vi "DRWM_SSF.vi"(0 "反应性in":dbl[](array[numeric]), 5 "SSF因子":cluster{"x":dbl, "y":dbl}[][](array[cluster]), 7 "P2信号":dbl[](array[numeric]), 9 "时间步长":sgl, 11 "通量in":dbl[](array[numeric]), 12 "首次调用？":bool) -> (4 "上下段通量索引":u16[](array[numeric]), 6 "DRWM开":bool, 8 "P2信号out":dbl[](array[numeric]), 10 "通量out":dbl[](array[numeric]), 14 "棒限":dbl[](array[numeric]), 15 "刻棒棒位":dbl)   [LabVIEW 2020]
uses:
  <vilib>/Analysis/baseanly.llb/Mean (DBL).vi
  <vilib>/Analysis/NI_AALBase.lvlib
panel:
  in  "DSF2合1":bool
  in  "上下段比值":dbl=0.0001 min=0.0001 max=100.0 step=0.0001 format="%0.2f"
  in  "修正因子选择":u16(ring) items=["C1", "C2", "C3", "C4", "C5", "C6", "C7", "C8", "C9", "10"]
  out "因子说明":string caption="修正因子文件说明："
  in  "因子棒名":string[](array[string])
  in  "底部棒位 (步)":dbl=5.0
  in  "触发准备":bool
  out "触发量稳定值":dbl
  in  "反应性触发选择":u16(ring) items=["电流1", "电流2"]
  out "触发量散度 (%)":dbl
  in  "触发量容限 (%)":dbl=10.0
  in  "反应性暂存":dbl[](array[numeric])
  in  "棒位暂存":dbl[](array[numeric])
  in  "触发方式":u16(ring)=3 items=["手动触发启动", "反应性触发启动", "棒位触发启动", "实时棒位无需触发"]
  in  "顶部棒位 (步)":dbl=225.0
  in  "棒速 (步/分钟)":dbl=72.0
  out "DRWM控制棒":dbl(slide) min=0.0 max=225.0 scale=0.0..225.0
  in  "开关":bool
  in  "上部探测器选择":u16(ring) items=["电流1", "电流2"]
  in  "下部探测器选择":u16(ring)=1 items=["电流1", "电流2"]
  in  "通量名称":string[](array[string])
  in  "P2名称":string[](array[string])
  in  "控制棒选择":i32(ring) items=["棒位D", "棒位C", "电压6"]
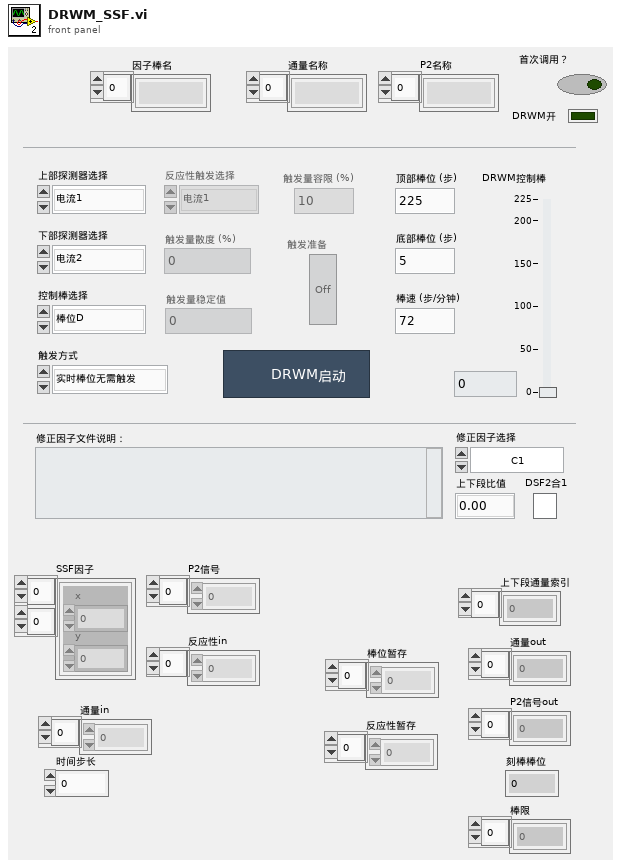
[diagram p1: front panel]
types:
  T1 = enum8{"Enabled", "Disabled", "Disabled and Grayed Out"}
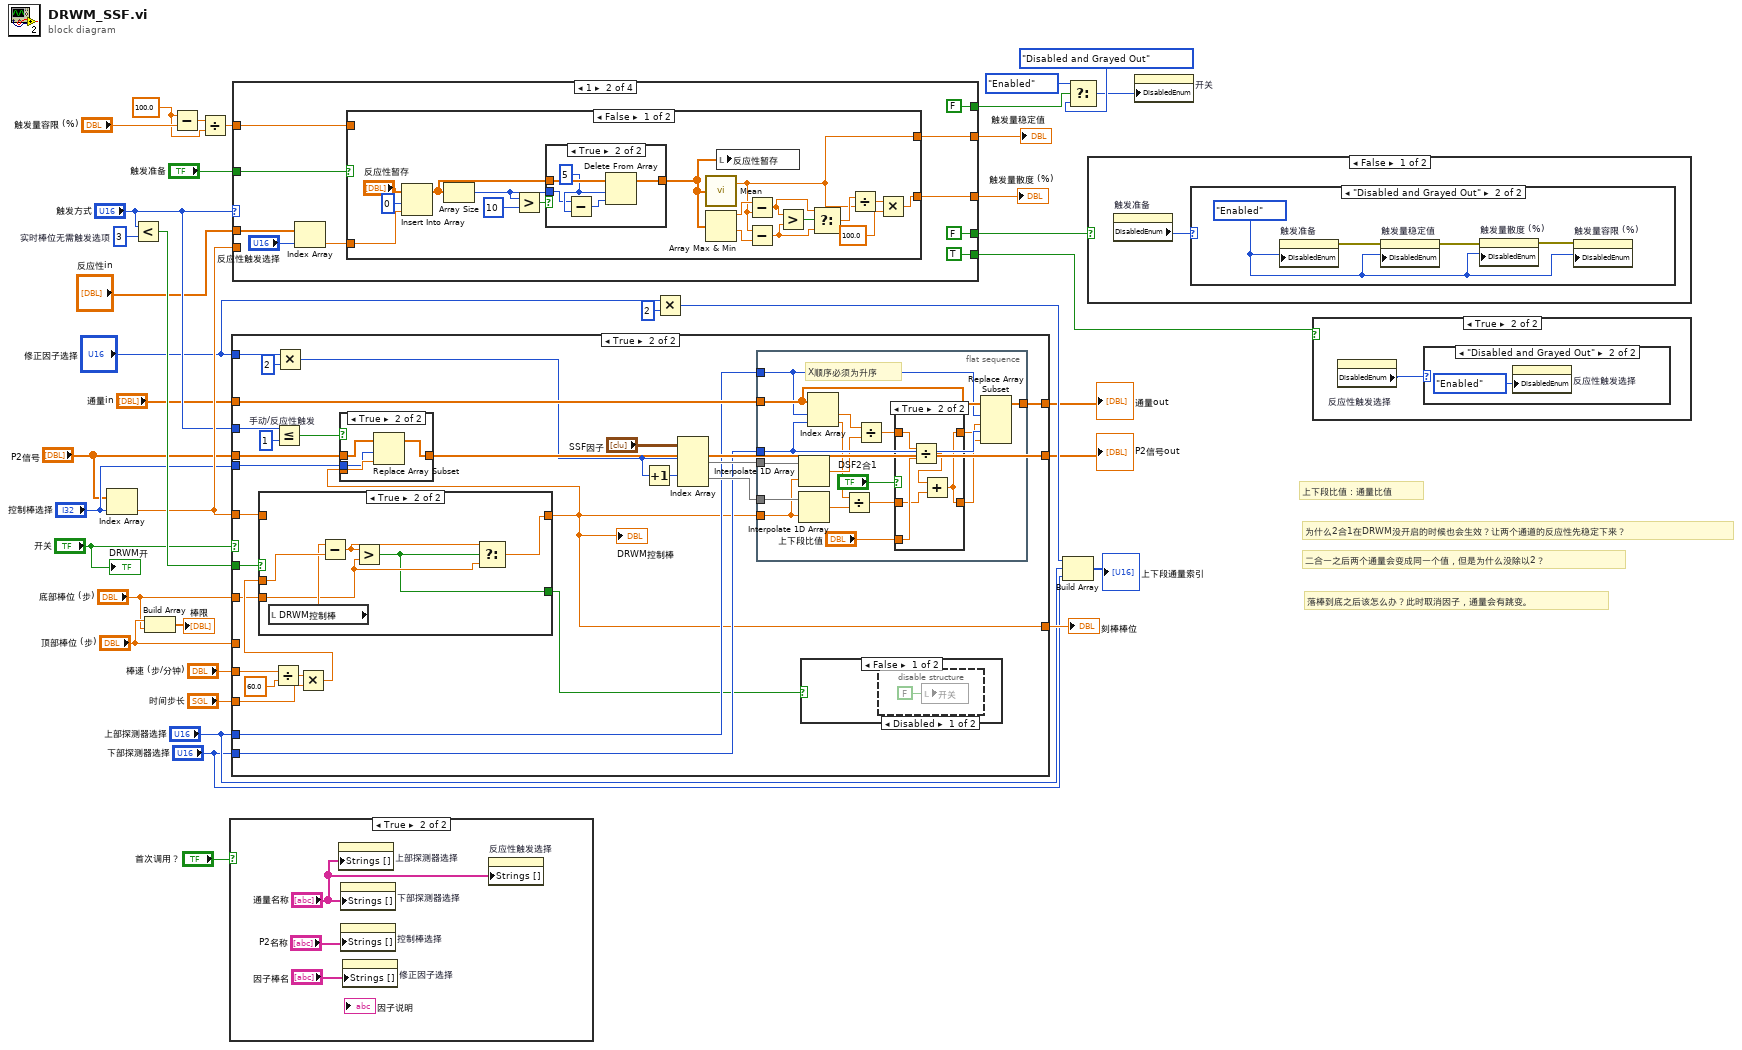
[diagram p0: block diagram]
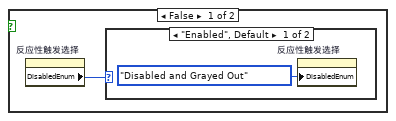
[diagram p2: hidden frame]
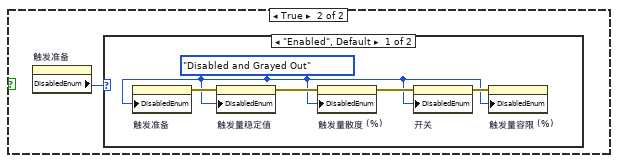
[diagram p6: hidden frame]
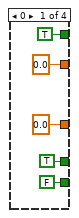
[diagram p8: hidden frame]
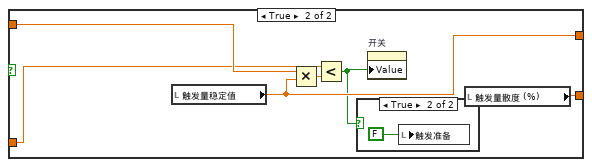
[diagram p10: hidden frame]
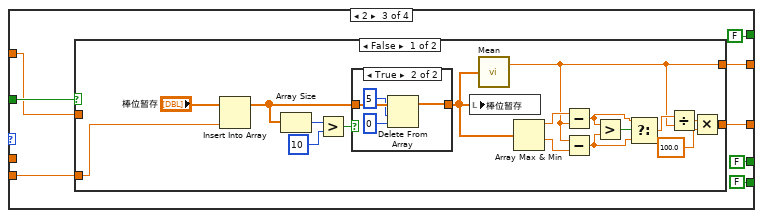
[diagram p12: hidden frame]
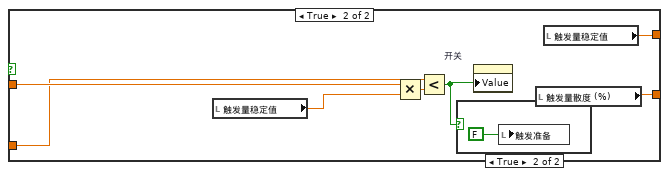
[diagram p14: hidden frame]
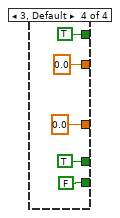
[diagram p16: hidden frame]
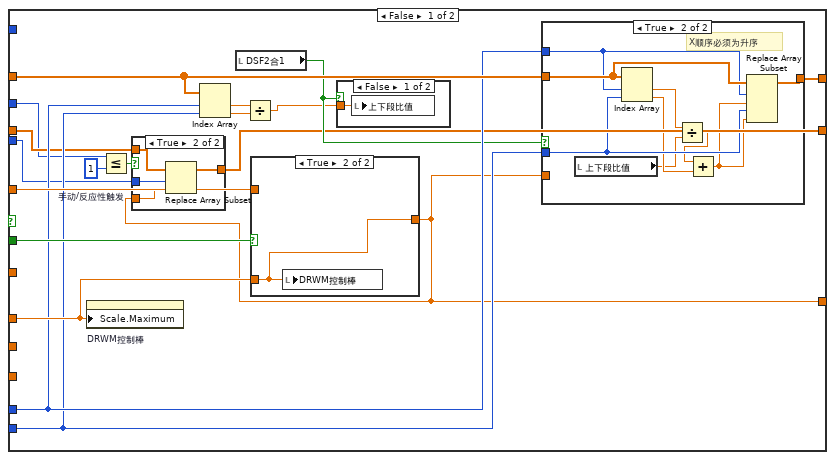
[diagram p17: hidden frame]
diagram:
  w31 = 100.0 ("x")
  w34 = u16 3  # 实时棒位无需触发选项
  # "落棒到底之后该怎么办？此时取消因子，通量会有跳变。"
  # "二合一之后两个通量会变成同一个值，但是为什么没除以2？"
  # "为什么2合1在DRWM没开启的时候也会生效？让两个通道的反应性先稳定下来？"
  # "上下段比值：通量比值"
  n1 = Index Array(array="P2信号", index="控制棒选择") -> (element=w30:dbl)
  n2 = Less?(x="触发方式", y=w34) -> (x < y?=w35:bool)
  n3 = Build Array("顶部棒位 (步)", "底部棒位 (步)") -> (→"棒限":dbl[])
  n4 = Subtract(x=w31, y="触发量容限 (%)") -> (x-y=w32:dbl)
  n5 = Divide(x=w32, y=w31) -> (x/y=w29:dbl)
  n6 = case shown="True" "首次调用？" {
    frame False {
    }
    frame True {
      n7 = property on="上部探测器选择" class="Ring (strict)"("Strings []"="通量名称") -> ()  [unwired: 2 in, 2 out]
      n8 = property on="下部探测器选择" class="Ring (strict)"("Strings []"="通量名称") -> ()  [unwired: 2 in, 2 out]
      n9 = property on="控制棒选择" class="Ring (strict)"("Strings []"="P2名称") -> ()  [unwired: 2 in, 2 out]
      n10 = property on="修正因子选择" class="Ring (strict)"("Strings []"="因子棒名") -> ()  [unwired: 2 in, 2 out]
      n11 = property on="反应性触发选择" class="Ring (strict)"("Strings []"="通量名称") -> ()  [unwired: 2 in, 2 out]
    }
  }
  n12 = case shown="True" "开关" {
    tunnel: "通量in" -> [w53 w103]
    tunnel: [w52 w102] -> w9
    tunnel: "棒速 (步/分钟)" -> [_ w98]
    tunnel: "时间步长" -> [_ w94]
    tunnel: "顶部棒位 (步)" -> [w56 _]
    tunnel: w35 -> [w57 w96]
    tunnel: w30 -> [w58 w95]
    tunnel: [w45 w78] -> w27
    tunnel: "P2信号" -> [w44 w88]
    tunnel: [w43 w87] -> w11
    tunnel: "触发方式" -> [w42 w91]
    tunnel: "控制棒选择" -> [w46 w86]
    tunnel: "底部棒位 (步)" -> [_ w85]
    tunnel: "修正因子选择" -> [_ w84]
    tunnel: "上部探测器选择" -> [w51 w80]
    tunnel: "下部探测器选择" -> [w50 w79]
    frame False {
      w48 = u16 1  # 手动/反应性触发
      n13 = property on="DRWM控制棒" class="Slide (strict)"("Scale.Maximum"=w56) -> ()  [unwired: 2 in, 2 out]
      n14 = Less Or Equal?(x=w42, y=w48) -> (x <= y?=w47:bool)
      n15 = Index Array(array=w53, index #1=w51, index #2=w50) -> (element #1=w55:dbl, element #2=w54:dbl)
      n16 = local read "DSF2合1"() -> (w49:bool)
      n17 = Divide(x=w55, y=w54) -> (x/y=w41:dbl)
      n18 = case shown="True" w57 {
        tunnel: [w75 w76] -> w45
        tunnel: w58 -> [w75 _]
        tunnel: w56 -> [_ w76]
        frame False {
          n19 = local write "DRWM控制棒"(w75) -> ()
        }
        frame True {
          n20 = local write "DRWM控制棒"(w76) -> ()
        }
      }
      n21 = case shown="True" w47 {
        tunnel: w44 -> [w59 w63]
        tunnel: [w59 w62] -> w43
        tunnel: w45 -> [_ w61]
        tunnel: w46 -> [_ w60]
        frame False {
        }
        frame True {
          n22 = Replace Array Subset(array=w63, new element=w61, index=w60) -> (w62:dbl[])
        }
      }
      n23 = case shown="False" w49 {
        tunnel: w41 -> [w74 _]
        frame False {
          n24 = local write "上下段比值"(w74) -> ()
        }
        frame True {
        }
      }
      n25 = case shown="True" w49 {
        tunnel: w53 -> [w64 w73]
        tunnel: [w64 w72] -> w52
        tunnel: w45 -> [_ _]
        tunnel: w51 -> [_ w71]
        tunnel: w50 -> [_ w70]
        frame False {
        }
        frame True {
          # "X顺序必须为升序"
          n26 = local read "上下段比值"() -> (w66:dbl)
          n27 = Index Array(array=w73, index #1=w71, index #2=w70) -> (element #1=w67:dbl, element #2=w68:dbl)
          n28 = Divide(x=w67, y=w66) -> (x/y=w65:dbl)
          n29 = Add(x=w65, y=w68) -> (x+y=w69:dbl)
          n30 = Replace Array Subset(array=w73, new element #1=w69, index #1=w71, new element #2=w69, index #2=w70) -> (w72:dbl[])
        }
      }
    }
    frame True {
      w90 = u16 1  # 手动/反应性触发
      n31 = Divide(x=w98, y=60.0) -> (x/y=w93:dbl)
      n32 = Less Or Equal?(x=w91, y=w90) -> (x <= y?=w89:bool)
      n33 = Multiply(x=w84, y=u16 2) -> (x*y=w81:u16)
      n34 = Multiply(x=w93, y=w94) -> (x*y=w92:dbl)
      n35 = case shown="True" w96 {
        tunnel: w95 -> [w134 _]
        tunnel: [w134 w137] -> w78
        tunnel: w92 -> [_ w142]
        tunnel: w85 -> [w136 w139]
        tunnel: [w135 w138] -> w77
        frame False {
          n36 = Greater?(x=w134, y=w136) -> (0:w135:bool)
        }
        frame True {
          n37 = local read "DRWM控制棒"() -> (w140:dbl)
          n38 = Subtract(x=w140, y=w142) -> (x-y=w141:dbl)
          n39 = Greater?(x=w141, y=w139) -> (0:w138:bool)
          n40 = Select(t=w141, s=w138, f=w139) -> (s? t:f=w137:dbl)
        }
      }
      "DRWM控制棒" <- w78
      n41 = case shown="True" w89 {
        tunnel: w88 -> [w129 w133]
        tunnel: [w129 w132] -> w87
        tunnel: w78 -> [_ w131]
        tunnel: w86 -> [_ w130]
        frame False {
        }
        frame True {
          n42 = Replace Array Subset(array=w133, new element=w131, index=w130) -> (w132:dbl[])
        }
      }
      n43 = Increment(x=w81) -> (x+1=w82:u16)
      n44 = Index Array(array="SSF因子", index (row) #1=w81, index (row) #2=w82) -> (element #1=w100:cluster{"x":dbl, "y":dbl}[], element #2=w99:cluster{"x":dbl, "y":dbl}[])  [unwired: 2 in]
      n45 = flat-sequence {
        tunnel: w103 -> [w121]
        tunnel: [w120] -> w102
        tunnel: w100 -> [w119]
        tunnel: w99 -> [w118]
        tunnel: w80 -> [w117]
        tunnel: w79 -> [w116]
        tunnel: w78 -> [w115]
        frame #0 {
          # "X顺序必须为升序"
          n46 = Interpolate 1D Array(1:w115, 2:w119) -> (0:w113:dbl)
          n47 = Interpolate 1D Array(1:w115, 2:w118) -> (0:w112:dbl)
          n48 = Index Array(array=w121, index #1=w117, index #2=w116) -> (element #1=w114:dbl, element #2=w111:dbl)
          n49 = Divide(x=w111, y=w112) -> (x/y=w109:dbl)
          n50 = Divide(x=w114, y=w113) -> (x/y=w110:dbl)
          n51 = case shown="True" "DSF2合1" {
            tunnel: w110 -> [w123 w128]
            tunnel: w109 -> [w122 w126]
            tunnel: [w122 w124] -> w108
            tunnel: [w123 w124] -> w107
            tunnel: "上下段比值" -> [_ w127]
            frame False {
            }
            frame True {
              n52 = Divide(x=w128, y=w127) -> (x/y=w125:dbl)
              n53 = Add(x=w125, y=w126) -> (x+y=w124:dbl)
            }
          }
          n54 = Replace Array Subset(array=w121, new element #1=w107, index #1=w117, new element #2=w108, index #2=w116) -> (w120:dbl[])
        }
      }
      n55 = case shown="False" w77 {
        frame False {
          n56 = disable-structure shown="Disabled" {
            frame Disabled {
              n57 = local write "开关"(FALSE ("开关")) -> ()
            }
            frame Enabled {
            }
          }
        }
        frame True {
        }
      }
    }
  }
  "通量out" <- w9
  "刻棒棒位" <- w27
  "P2信号out" <- w11
  n58 = case shown="1" "触发方式" {
    tunnel: w30 -> [_ _ w196 _]
    tunnel: w29 -> [_ w151 w193 _]
    tunnel: "反应性in" -> [_ w153 _ _]
    tunnel: [0.0 ("触发量散度%") w157 w195 0.0] -> w28
    tunnel: [0.0 ("mean") w156 w192 0.0 ("触发量稳定值")] -> w26
    tunnel: "触发准备" -> [_ w152 w194 _]
    tunnel: [TRUE FALSE FALSE TRUE] -> w24
    tunnel: [FALSE TRUE FALSE FALSE] -> w23
    tunnel: [TRUE FALSE FALSE TRUE] -> w4
    frame 0 {
    }
    frame 1 {
      n59 = Index Array(array=w153, index="反应性触发选择") -> (element=w154:dbl)
      n60 = case shown="False" w152 {
        tunnel: [w160 w187] -> w157
        tunnel: [w159 w185] -> w156
        tunnel: w154 -> [w158 w182]
        tunnel: w151 -> [_ w183]
        frame False {
          n61 = Insert Into Array(array="反应性暂存", index=0 ("索引"), new element=w158) -> (w172:dbl[])
          n62 = Array Size(array=w172) -> (size(s)=w170:i32)
          n63 = Greater?(x=w170, y=10) -> (0:w175:bool)
          n64 = case shown="True" w175 {
            tunnel: w172 -> [w176 w180]
            tunnel: [w176 w181] -> w171
            tunnel: w170 -> [_ w178]
            frame False {
            }
            frame True {
              w179 = 5 ("长度")
              n65 = Subtract(x=w178, y=w179) -> (x-y=w177:i32)
              n66 = Delete From Array(array=w180, length=w179, index=w177) -> (array with subset deleted=w181:dbl[])  [unwired: 1 out]
            }
          }
          n67 = call-poly <vilib>:"Mean.vi"("X"=w171) -> ("mean"=w159:dbl)  [unwired: 1 out]
          n68 = Array Max & Min(array=w171) -> (max value=w168:dbl, min value=w167:dbl)  [unwired: 2 out]
          n69 = local write "反应性暂存"(w171) -> ()
          n70 = Subtract(x=w168, y=w159) -> (x-y=w165:dbl)
          n71 = Subtract(x=w159, y=w167) -> (x-y=w164:dbl)
          n72 = Greater?(x=w165, y=w164) -> (0:w166:bool)
          n73 = Select(t=w165, s=w166, f=w164) -> (s? t:f=w163:dbl)
          n74 = Divide(x=w163, y=w159) -> (x/y=w162:dbl)
          n75 = Multiply(x=w162, y=100.0) -> (x*y=w160:dbl)
        }
        frame True {
          n76 = local read "触发量稳定值"() -> (w185:dbl)
          n77 = Multiply(x=w183, y=w185) -> (x*y=w186:dbl)
          n78 = Less?(x=w182, y=w186) -> (x < y?=w184:bool)
          n79 = case shown="True" w184 {
            frame False {
            }
            frame True {
              n80 = local write "触发准备"(FALSE ("触发准备")) -> ()
            }
          }
          n81 = property on="开关" class="Bool (strict)"("Value"=w184) -> ()  [unwired: 2 in, 2 out]
          n82 = local read "触发量散度 (%)"() -> (w187:dbl)
        }
      }
    }
    frame 2 {
      n83 = case shown="False" w194 {
        tunnel: w196 -> [w208 w219]
        tunnel: [w198 w224] -> w195
        tunnel: w193 -> [_ w222]
        tunnel: [w197 w220] -> w192
        frame False {
          n84 = Insert Into Array(array="棒位暂存", new element=w208) -> (w212:dbl[])  [unwired: 1 in]
          n85 = Array Size(array=w212) -> (size(s)=w210:i32)
          n86 = Greater?(x=w210, y=10) -> (0:w213:bool)
          n87 = case shown="True" w213 {
            tunnel: w212 -> [w214 w217]
            tunnel: [w214 w218] -> w204
            frame False {
            }
            frame True {
              n88 = Delete From Array(array=w217, length=5 ("长度"), index=0 ("索引")) -> (array with subset deleted=w218:dbl[])  [unwired: 1 out]
            }
          }
          n89 = local write "棒位暂存"(w204) -> ()
          n90 = call-poly <vilib>:"Mean.vi"("X"=w204) -> ("mean"=w197:dbl)  [unwired: 1 out]
          n91 = Array Max & Min(array=w204) -> (max value=w203:dbl, min value=w207:dbl)  [unwired: 2 out]
          n92 = Subtract(x=w203, y=w197) -> (x-y=w202:dbl)
          n93 = Subtract(x=w197, y=w207) -> (x-y=w205:dbl)
          n94 = Greater?(x=w202, y=w205) -> (0:w206:bool)
          n95 = Select(t=w202, s=w206, f=w205) -> (s? t:f=w199:dbl)
          n96 = Divide(x=w199, y=w197) -> (x/y=w201:dbl)
          n97 = Multiply(x=w201, y=100.0) -> (x*y=w198:dbl)
        }
        frame True {
          n98 = local read "触发量稳定值"() -> (w223:dbl)
          n99 = Multiply(x=w222, y=w223) -> (x*y=w225:dbl)
          n100 = Less?(x=w219, y=w225) -> (x < y?=w221:bool)
          n101 = case shown="True" w221 {
            frame False {
            }
            frame True {
              n102 = local write "触发准备"(FALSE ("触发准备")) -> ()
            }
          }
          n103 = property on="开关" class="Bool (strict)"("Value"=w221) -> ()  [unwired: 2 in, 2 out]
          n104 = local read "触发量散度 (%)"() -> (w224:dbl)
          n105 = local read "触发量稳定值"() -> (w220:dbl)
        }
      }
    }
    frame 3, Default {
    }
  }
  "触发量散度 (%)" <- w28
  "触发量稳定值" <- w26
  n106 = Multiply(x="修正因子选择", y=u16 2) -> (x*y=w13:u16)
  n107 = Build Array(w13, "上部探测器选择", "下部探测器选择") -> (→"上下段通量索引":u16[])
  n108 = Select(t=T1."Enabled" ("禁用"), s=w4, f=T1."Disabled and Grayed Out" ("禁用")) -> (s? t:f=w1:T1)
  n109 = case shown="False" w24 {
    frame False {
      n110 = property on="触发准备" class="Bool (strict)"() -> ("DisabledEnum"=w232:T1)  [unwired: 2 in, 2 out]
      n111 = case shown="\"Disabled and Grayed Out\"" w232 {
        frame "Enabled", Default {
        }
        frame "Disabled and Grayed Out" {
          w234 = T1."Enabled" ("禁用")
          n112 = property on="触发准备" class="Bool (strict)"("DisabledEnum"=w234) -> (error out=w236:errorcluster)  [unwired: 2 in, 1 out]
          n113 = property on="触发量稳定值" class="DigNum (strict)"(error in=w236, "DisabledEnum"=w234) -> (error out=w235:errorcluster)  [unwired: 1 in, 1 out]
          n114 = property on="触发量散度 (%)" class="DigNum (strict)"(error in=w235, "DisabledEnum"=w234) -> (error out=w233:errorcluster)  [unwired: 1 in, 1 out]
          n115 = property on="触发量容限 (%)" class="DigNum (strict)"(error in=w233, "DisabledEnum"=w234) -> ()  [unwired: 1 in, 2 out]
        }
      }
    }
    frame True {
      n116 = property on="触发准备" class="Bool (strict)"() -> ("DisabledEnum"=w237:T1)  [unwired: 2 in, 2 out]
      n117 = case shown="\"Enabled\", Default" w237 {
        frame "Enabled", Default {
          w238 = T1."Disabled and Grayed Out" ("禁用")
          n118 = property on="触发准备" class="Bool (strict)"("DisabledEnum"=w238) -> (error out=w241:errorcluster)  [unwired: 2 in, 1 out]
          n119 = property on="触发量稳定值" class="DigNum (strict)"(error in=w241, "DisabledEnum"=w238) -> (error out=w242:errorcluster)  [unwired: 1 in, 1 out]
          n120 = property on="触发量散度 (%)" class="DigNum (strict)"(error in=w242, "DisabledEnum"=w238) -> (error out=w240:errorcluster)  [unwired: 1 in, 1 out]
          n121 = property on="开关" class="Bool (strict)"(error in=w240, "DisabledEnum"=w238) -> (error out=w239:errorcluster)  [unwired: 1 in, 1 out]
          n122 = property on="触发量容限 (%)" class="DigNum (strict)"(error in=w239, "DisabledEnum"=w238) -> ()  [unwired: 1 in, 2 out]
        }
        frame "Disabled and Grayed Out" {
        }
      }
    }
  }
  n123 = property on="开关" class="Bool (strict)"("DisabledEnum"=w1) -> ()  [unwired: 2 in, 2 out]
  n124 = case shown="True" w23 {
    frame False {
      n125 = property on="反应性触发选择" class="Ring (strict)"() -> ("DisabledEnum"=w243:T1)  [unwired: 2 in, 2 out]
      n126 = case shown="\"Enabled\", Default" w243 {
        frame "Enabled", Default {
          n127 = property on="反应性触发选择" class="Ring (strict)"("DisabledEnum"=T1."Disabled and Grayed Out" ("禁用")) -> ()  [unwired: 2 in, 2 out]
        }
        frame "Disabled and Grayed Out" {
        }
      }
    }
    frame True {
      n128 = property on="反应性触发选择" class="Ring (strict)"() -> ("DisabledEnum"=w245:T1)  [unwired: 2 in, 2 out]
      n129 = case shown="\"Disabled and Grayed Out\"" w245 {
        frame "Enabled", Default {
        }
        frame "Disabled and Grayed Out" {
          n130 = property on="反应性触发选择" class="Ring (strict)"("DisabledEnum"=T1."Enabled" ("禁用")) -> ()  [unwired: 2 in, 2 out]
        }
      }
    }
  }
  "DRWM开" <- "开关"
